vi "Read Key.vi"(7 "section":string, 8 "error in (no error)":errorcluster, 9 "default value":string, 10 "key":string) -> (0 "error out":errorcluster, 2 "value":string)   [LabVIEW 2020, in "Configuration Manager.lvclass"]
uses:
  Configuration Manager.lvclass
  <vilib>/Utility/config.llb/Read Key (String).vi
  <vilib>/Utility/config.llb/Write Key (Boolean).vi
  <vilib>/Utility/config.llb/NI_LVConfig.lvlib
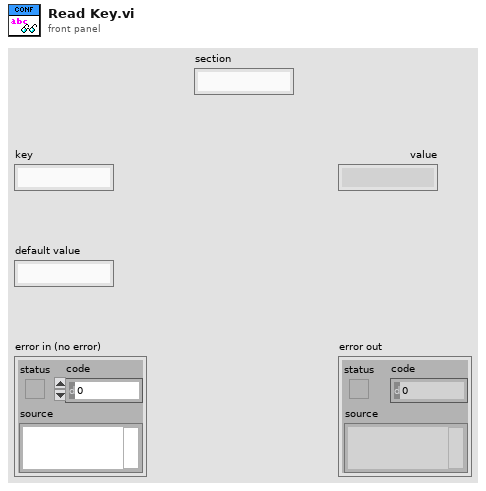
[diagram p1: front panel]
types:
  T1 = typedef "NI_LVConfig.lvlib/Config Data RefNum.ctl" = refnum<k1>
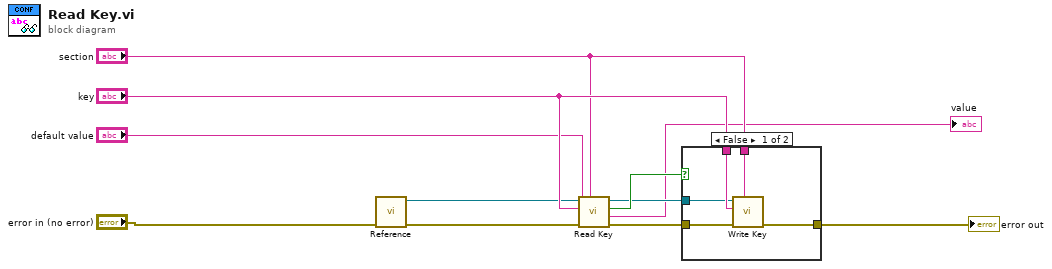
[diagram p0: block diagram]
diagram:
  n1 = call "Reference.vi"("error in (no error)"="error in (no error)") -> ("error out"=w10:errorcluster, "Refnum out"=w1:T1)  [unwired: 9 in]
  n2 = call-poly <vilib>:"Read Key.vi"("section"="section", "error in (no error)"=w10, "default value"="default value", "key"="key", "refnum"=w1) -> ("error out"=w9:errorcluster, "value"=→"value":string, "found?"=w7:bool, "refnum out"=w4:T1)  [unwired: 3 in]
  n3 = case shown="False" w7 {
    tunnel: w9 -> [w16 w17]
    tunnel: "key" -> [w15 _]
    tunnel: "section" -> [w14 _]
    tunnel: [w13 w17] -> w8
    tunnel: w4 -> [w12 _]
    frame False {
      n4 = call-poly <vilib>:"Write Key.vi"("section"=w14, "error in (no error)"=w16, "key"=w15, "refnum"=w12) -> ("error out"=w13:errorcluster)  [unwired: 5 in, 2 out]
    }
    frame True {
    }
  }
  "error out" <- w8
